vi "Insight_FFT.vi"(8 "error in (no error)":errorcluster, 9 "FFT Parameters":T1={"Window"=enum."Hamming", "Gaussian Edge Roll-off (dB)"=10.0, "Zero-Pad the FFT?"=FALSE, "Powers of 2 higher"=1}, 10 "Data":dbl[](array[numeric])) -> (0 "error out":errorcluster, 1 "Size of FFT":i32, 2 "Power Spectrum":dbl[](array[numeric]))   [LabVIEW 2011]
doc: "Insight Photonic Solutions\n\nThis VI calculates Power Spectrum of an input Data array. The FFT may be processed with a variety of window functions, including a Gaussian window. To apply the Gaussian, you need to specify how much the Gaussian rolls off at the edges of the data set. Finally, you can optionally choose to perform zero-padding up to the next higher power of 2, both to expedite the FFT and to increase the bin resolution.\n\nPower Spectrum = 20*Log(Amplitude), in dB\n\nver 1.0 - original release"
uses:
  <vilib>/Analysis/2dsp.llb/Real FFT.vi
  <vilib>/Analysis/4window.llb/Hanning Window (DBL).vi
  <vilib>/Analysis/4window.llb/Blackman-Harris Window (DBL).vi
  <vilib>/Analysis/4window.llb/Hamming Window (DBL).vi
  <vilib>/Analysis/4window.llb/Blackman Window (DBL).vi
  <vilib>/Analysis/4window.llb/Gaussian Window (DBL).vi
  <vilib>/Analysis/NI_AALPro.lvlib
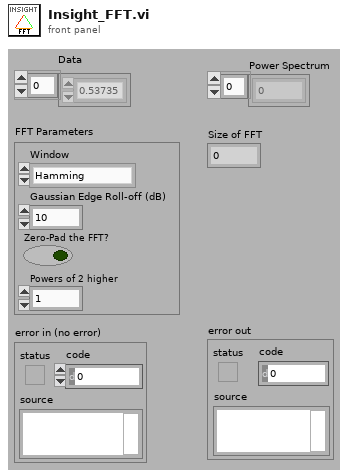
[diagram p1: front panel]
types:
  T1 = cluster{"Window":enum16{"Rectangular", "Hanning", "Hamming", "Blackman", "Blackman-Harris", "Gaussian+Hamming", "Gaussian+B-H"}, "Gaussian Edge Roll-off (dB)":dbl, "Zero-Pad the FFT?":bool, "Powers of 2 higher":i32}
  T2 = enum16{"Rectangular", "Hanning", "Hamming", "Blackman", "Blackman-Harris", "Gaussian+Hamming", "Gaussian+B-H"}
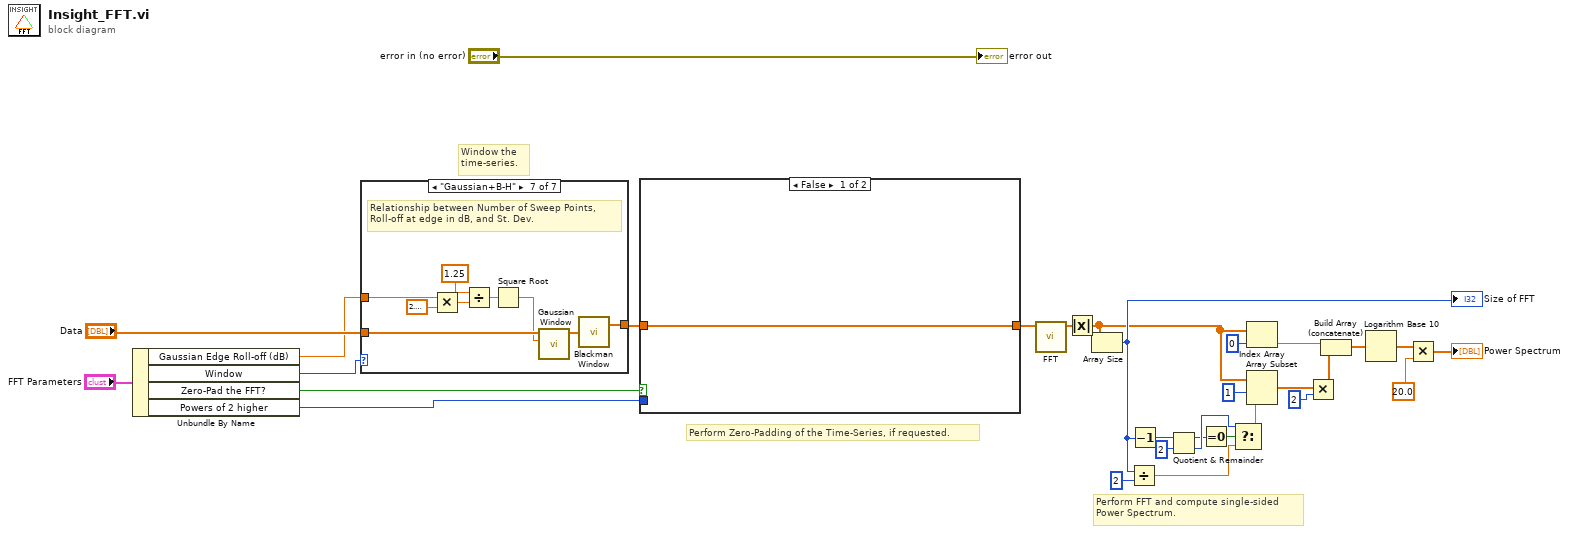
[diagram p0: block diagram]
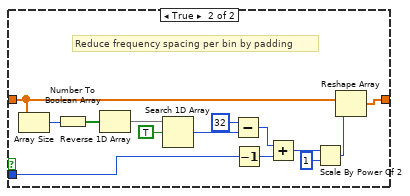
[diagram p2: hidden frame]
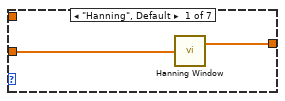
[diagram p3: hidden frame]
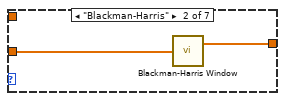
[diagram p4: hidden frame]
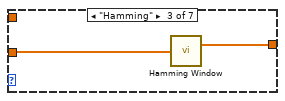
[diagram p5: hidden frame]
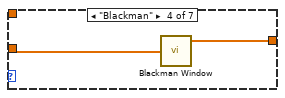
[diagram p6: hidden frame]
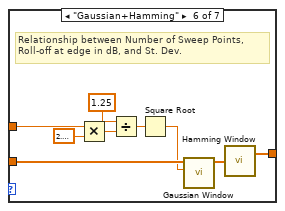
[diagram p8: hidden frame]
diagram:
  # "Perform FFT and compute single-sided\nPower Spectrum."
  # "Window the \ntime-series."
  # "Perform Zero-Padding of the Time-Series, if requested."
  n1 = Unbundle By Name("FFT Parameters") -> ("Gaussian Edge Roll-off (dB)"=w1:dbl, "Window"=w4:T2, "Zero-Pad the FFT?"=w3:bool, "Powers of 2 higher"=w2:i32)
  n2 = case shown="\"Gaussian+B-H\"" w4 {
    tunnel: [w32 w34 w35 w37 w39 w48 w56] -> w20
    tunnel: "Data" -> [w31 w33 w36 w38 w39 w41 w50]
    tunnel: w1 -> [_ _ _ _ _ w42 w51]
    frame "Hanning", Default {
      n3 = call-poly <vilib>:"Hanning Window.vi"("X"=w31) -> ("Windowed X"=w32:dbl[])  [unwired: 1 out]
    }
    frame "Blackman-Harris" {
      n4 = call-poly <vilib>:"Blackman-Harris Window.vi"("X"=w33) -> ("Windowed X"=w34:dbl[])  [unwired: 1 out]
    }
    frame "Hamming" {
      n5 = call-poly <vilib>:"Hamming Window.vi"("X"=w36) -> ("Windowed X"=w35:dbl[])  [unwired: 1 out]
    }
    frame "Blackman" {
      n6 = call-poly <vilib>:"Blackman Window.vi"("X"=w38) -> ("Windowed X"=w37:dbl[])  [unwired: 1 out]
    }
    frame "Rectangular" {
    }
    frame "Gaussian+Hamming" {
      # "Relationship between Number of Sweep Points,\nRoll-off at edge in dB, and St. Dev."
      n7 = Multiply(x=w42, y=2.302585092994046) -> (x*y=w45:dbl)
      n8 = Divide(x=1.25, y=w45) -> (x/y=w43:dbl)
      n9 = Square Root(x=w43) -> (sqrt(x)=w40:dbl)
      n10 = call-poly <vilib>:"Gaussian Window.vi"("standard deviation"=w40, "X"=w41) -> ("Windowed X"=w47:dbl[])  [unwired: 8 in, 1 out]
      n11 = call-poly <vilib>:"Hamming Window.vi"("X"=w47) -> ("Windowed X"=w48:dbl[])  [unwired: 1 out]
    }
    frame "Gaussian+B-H" {
      # "Relationship between Number of Sweep Points,\nRoll-off at edge in dB, and St. Dev."
      n12 = Multiply(x=w51, y=2.302585092994046) -> (x*y=w54:dbl)
      n13 = Divide(x=1.25, y=w54) -> (x/y=w52:dbl)
      n14 = Square Root(x=w52) -> (sqrt(x)=w49:dbl)
      n15 = call-poly <vilib>:"Gaussian Window.vi"("standard deviation"=w49, "X"=w50) -> ("Windowed X"=w57:dbl[])  [unwired: 8 in, 1 out]
      n16 = call-poly <vilib>:"Blackman Window.vi"("X"=w57) -> ("Windowed X"=w56:dbl[])  [unwired: 1 out]
    }
  }
  n17 = case shown="False" w3 {
    tunnel: [w58 w72] -> w19
    tunnel: w2 -> [_ w66]
    tunnel: w20 -> [w58 w62]
    frame False {
    }
    frame True {
      # "Reduce frequency spacing per bin by padding"
      n18 = Array Size(array=w62) -> (size(s)=w60:i32)
      n19 = Number To Boolean Array(number=w60) -> (Boolean array=w70:bool[])
      n20 = Reverse 1D Array(array=w70) -> (reversed array=w69:bool[])
      n21 = Search 1D Array(1D array=w69, element=TRUE) -> (index of element=w68:i32)  [unwired: 1 in]
      n22 = Subtract(x=32, y=w68) -> (x-y=w65:i32)
      n23 = Decrement(x=w66) -> (x-1=w61:i32)
      n24 = Add(x=w65, y=w61) -> (x+y=w64:i32)
      n25 = Scale By Power Of 2(n=w64, x=1) -> (x*2^n=w59:i32)
      n26 = Reshape Array(w62, w59) -> (w72:dbl[])
    }
  }
  n27 = call-poly <vilib>:"FFT.vi"("X"=w19) -> ("FFT {X}"=w29:cdb[])  [unwired: 9 in, 1 out]
  n28 = Absolute Value(x=w29) -> (abs(x)=w7:dbl[])
  n29 = Array Size(array=w7) -> (size(s)=w10:i32)
  "Size of FFT" <- w10
  n30 = Divide(x=w10, y=2) -> (x/y=w18:dbl)
  n31 = Decrement(x=w10) -> (x-1=w12:i32)
  n32 = Quotient & Remainder(x=w12, y=2) -> (x-y*floor(x/y)=w14:i32, floor(x/y)=w16:i32)
  n33 = Equal To 0?(x=w14) -> (x = 0?=w15:bool)
  n34 = Select(t=w16, s=w15, f=w18) -> (s? t:f=w11:dbl)
  n35 = Index Array(array=w7, index=0) -> (element=w26:dbl)
  n36 = Array Subset(array=w7, index=1, length=w11) -> (w25:dbl[])
  n37 = Multiply(x=w25, y=2) -> (x*y=w23:dbl[])
  n38 = Build Array (concatenate)(w26, w23) -> (w9:dbl[])
  n39 = Logarithm Base 10(1:w9) -> (0:w22:dbl[])
  n40 = Multiply(x=w22, y=20.0) -> (x*y=→"Power Spectrum":dbl[])
  "error out" <- "error in (no error)"
